vi "LDA_Align_PN.vi"() -> (0 "Beam Data":T1={"Vg1 (Green 1 dir. vect.)"=[0.059117350659853476, -0.996541267827751, 0.05840068807144843], "Vg2  (Green 2 dir. vect.)"=[-0.05232536310393669, -0.9971561380468801, -0.054237373935992664], "Vb1 (Blue 1 dir. vect.)"=[-0.052923229613528855, -0.9969242065933935, 0.057803616456121795], "Vb2 (Blue 1 dir. vect.)"=[0.05971521716944564, -0.9967731992812374, -0.05364030232066602], "Porb (Orb XYZ posn. forced coplanar)"=[2201.0738225655555, -1199.3737231995547, 269.758310600838], "Porb (Orb XYZ posn. - allow skew)"=[2200.796256301178, -1199.3740953152687, 270.0329332816893], "Orb posn. uncertainty, +/- dx, dy, dz"=[0.13878313218879157, 0.00018605785703584843, 0.13731134042564008], "Vp (Actual Probe dir. vect)"=[0.003406702197773746, -0.9999920168246164, 0.0020882210543692924], "Yaw (deg)"=89.80480953887573, "Pitch (deg)"=0.11964634006213794, "In-Plane Roll (deg)"=45.305328966424156, "Beam Half Angle (deg)"=4.544091484248422, "B1 Close P11"=[0.0, 0.0, 0.0], "B1 Far P12"=[2158.01, -491.04, 229.28], "B2 Close P22"=[2158.01, -491.04, 229.28], "B2 Far P21"=[2158.01, -491.04, 229.28], "Projected Roll (deg)"=0.0, "Green Velocity Vector"=[0.0, 0.0, 0.0], "Blue Velocity Vector"=[0.0, 0.0, 0.0], "Probe is facing...."="-", "Calculation Method"=""} {"Vp (Actual Probe dir. vect)" format="%#_6f"; "Vg2  (Green 2 dir. vect.)" format="%#_6f"; "Vg1 (Green 1 dir. vect.)" format="%#_6f"})   [LabVIEW 2011]
uses:
  Controls/LDA_Beam_Cluster.ctl
  Gen Trav/Route mapping/Axis.ctl
  Controls/User_Specific_mode.ctl
  Globals/Constants_global.vi
  Globals/Trav_pos_global.vi
  Globals/LDA_meas_global_1.vi
  Utilities/Email_transfer_global.vi
panel:
  # "Run this Vi again if you taught the laser positions but something went wrong after that"
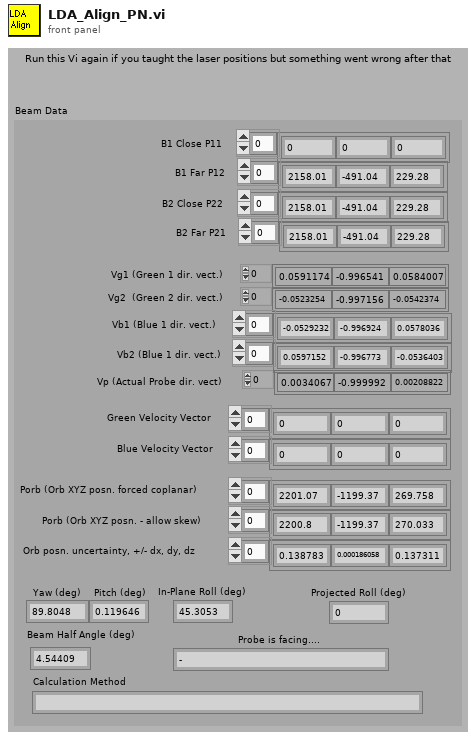
[diagram p1: front panel]
types:
  T1 = typedef "LDA_Beam_Cluster.ctl" = cluster{"Vg1 (Green 1 dir. vect.)":dbl[], "Vg2  (Green 2 dir. vect.)":dbl[], "Vb1 (Blue 1 dir. vect.)":dbl[], "Vb2 (Blue 1 dir. vect.)":dbl[], "Porb (Orb XYZ posn. forced coplanar)":dbl[], "Porb (Orb XYZ posn. - allow skew)":dbl[], "Orb posn. uncertainty, +/- dx, dy, dz":dbl[], "Vp (Actual Probe dir. vect)":dbl[], "Yaw (deg)":dbl, "Pitch (deg)":dbl, "In-Plane Roll (deg)":dbl, "Beam Half Angle (deg)":dbl, "B1 Close P11":dbl[], "B1 Far P12":dbl[], "B2 Close P22":dbl[], "B2 Far P21":dbl[], "Projected Roll (deg)":dbl, "Green Velocity Vector":dbl[], "Blue Velocity Vector":dbl[], "Probe is facing....":string, "Calculation Method":string}
  T2 = typedef "Axis.ctl" = enum16{"X Axis", "X Axis -ve", "Y Axis", "Y Axis -ve", "Z Axis", "Z Axis -ve"}
  T3 = typedef "User_Specific_mode.ctl" = enum16{"Check VI only", "Run VI"}
  T4 = enum16{"Load setup from excel file", "Save setup to excel file"}
  T5 = enum16{"Load From Excel File", "Save to Excel File"}
  T6 = cluster{"second":i32, "minute":i32, "hour":i32, "day of month":i32, "month":i32, "year":i32, "day of week":i32, "day of year":i32, "is DST":i32}
  T7 = typedef "Multi_Run_Status.ctl" = enum16{"Continue", "Jump to Next Point", "Jump to Next Row", "Jump To Fall Back", "Terminate Run"}
  T8 = cluster{"path":path, "data":string, "binary":bool, "MIME content-type \n(application/octet-stream)":string}[]
  T9 = cluster{"path":path, "data":string, "binary":bool, "MIME content-type \n(application/octet-stream)":string}
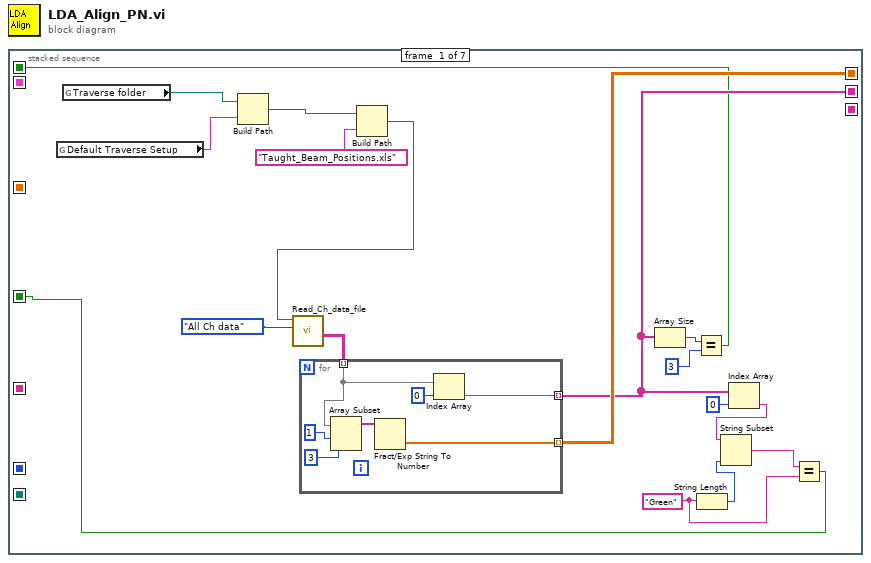
[diagram p0: block diagram]
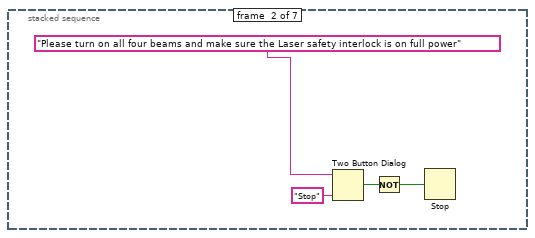
[diagram p2: hidden frame]
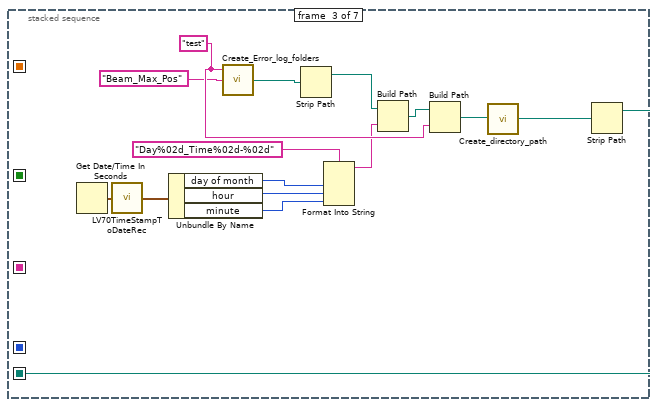
[diagram p3: hidden frame]
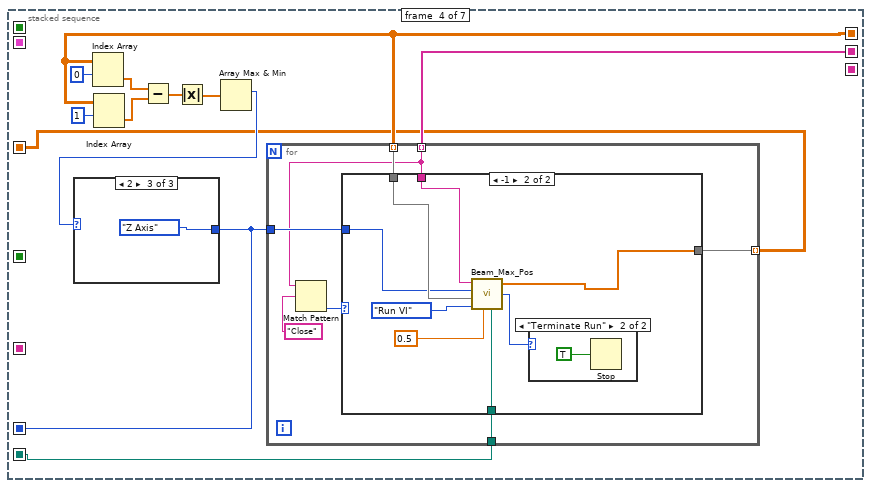
[diagram p4: hidden frame]
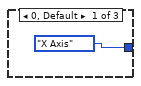
[diagram p5: hidden frame]
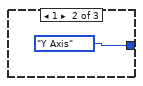
[diagram p6: hidden frame]
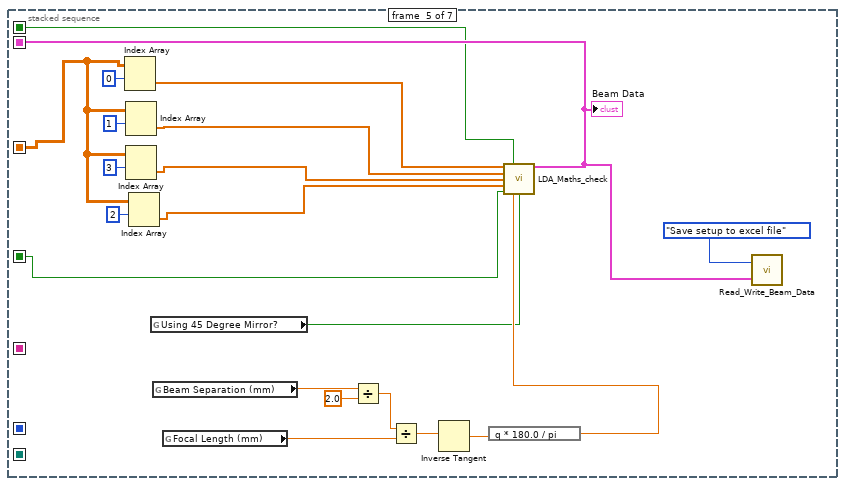
[diagram p9: hidden frame]
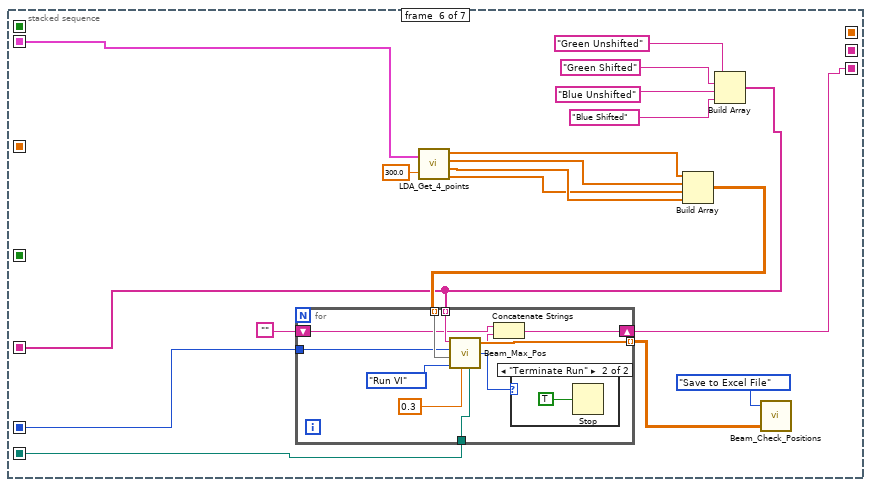
[diagram p10: hidden frame]
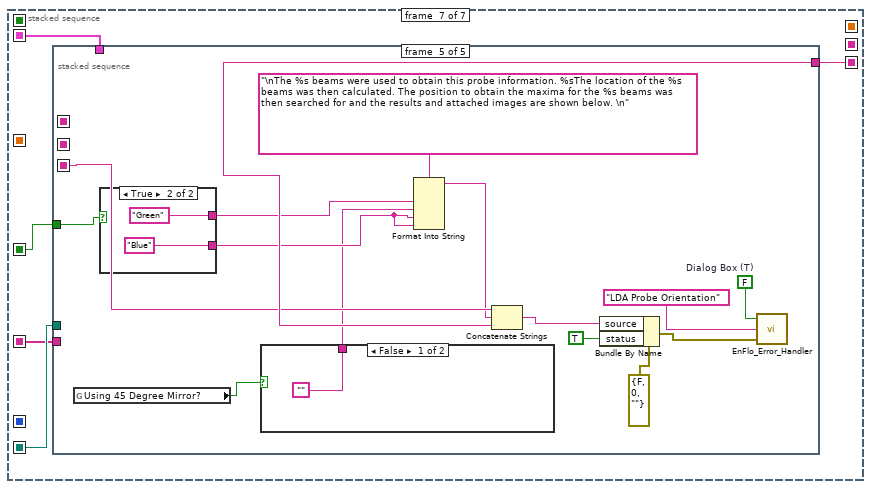
[diagram p12: hidden frame]
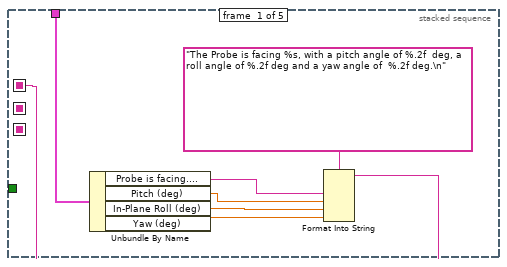
[diagram p13: hidden frame]
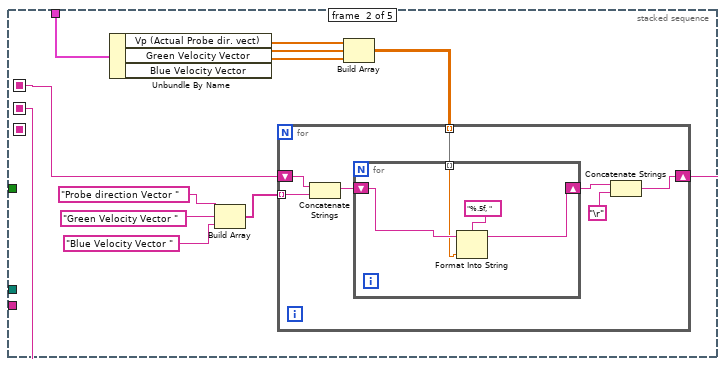
[diagram p14: hidden frame]
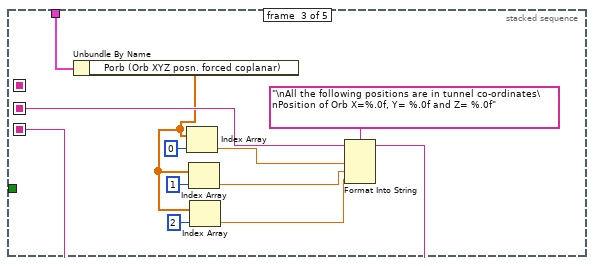
[diagram p15: hidden frame]
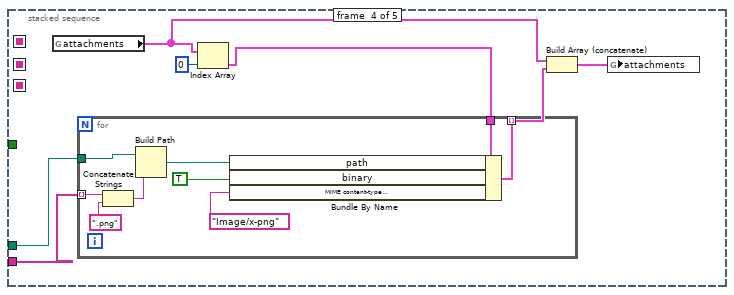
[diagram p16: hidden frame]
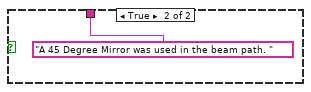
[diagram p17: hidden frame]
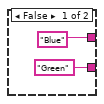
[diagram p18: hidden frame]
diagram:
  n1 = stacked-sequence {
    seq-local: [_ _ _ _ w96 _ _] -> [_ _ _ _ _ w115 w129]
    seq-local: [w12 _ _ _ _ _ _] -> [_ _ _ w53 _ _ _]
    seq-local: [w4 _ _ _ _ _ _] -> [_ _ _ w56 _ _ _]
    seq-local: [_ _ _ w47 _ _ _] -> [_ _ _ _ w84 _ _]
    seq-local: [_ _ w32 _ _ _ _] -> [_ _ _ w46 _ w113 w132]
    seq-local: [_ _ _ w45 _ _ _] -> [_ _ _ _ _ w114 _]
    seq-local: [_ _ _ _ _ w111 _] -> [_ _ _ _ _ _ w131]
    seq-local: [_ _ _ _ _ w109 _] -> [_ _ _ _ _ _ w130]
    seq-local: [w5 _ _ _ _ _ _] -> [_ _ _ _ w78 _ w128]
    seq-local: [w1 _ _ _ _ _ _] -> [_ _ _ _ w77 _ _]
    frame #0 {
      w6 = "Green"
      n2 = global read "Trav_pos_global.vi" "Default Traverse Setup"() -> (w16:string)
      n3 = global read "Constants_global.vi" "Traverse folder"() -> (w18:path)
      n4 = Build Path(base path=w18, name or relative path=w16) -> (appended path=w17:path)
      n5 = Build Path(base path=w17, name or relative path="Taught_Beam_Positions.xls" ("Substring")) -> (appended path=w11:path)
      n6 = call "Read_Ch_data_file.vi"("Output"=enum16{"All Ch data", "The last few rows"}."All Ch data", "Filename"=w11) -> ("Channel Values"=w14:string[][])  [unwired: 3 in, 4 out]
      n7 = for {
        tunnel: w14 -> [w21] mode=indexing
        tunnel: [w23] -> w12 mode=indexing
        tunnel: [w19] -> w4 mode=indexing
        n8 = Array Subset(array=w21, index=1 ("Array Index"), length=3) -> (w24:string[])
        n9 = Fract/Exp String To Number(string=w24) -> (number=w23:dbl[])  [unwired: 4 out]
        n10 = Index Array(array=w21, index=0) -> (element=w19:string)
      }
      n11 = Array Size(array=w4) -> (size(s)=w3:i32)
      n12 = Equal?(x=w3, y=3) -> (x = y?=w1:bool)
      n13 = String Length(string=w6) -> (length=w8:i32)
      n14 = Index Array(array=w4, index=0) -> (element=w9:string)
      n15 = String Subset(string=w9, length (rest)=w8) -> (substring=w7:string)  [unwired: 1 out]
      n16 = Equal?(x=w7, y=w6) -> (x = y?=w5:bool)
    }
    frame #1 {
      n17 = Two Button Dialog(message="Please turn on all four beams and make sure the Laser safety interlock is on full power", 1:"Stop" ("F button name (\"Cancel\")")) -> (T button?=w28:bool)  [unwired: 1 out]
      n18 = Not(x=w28) -> (.not. x?=w27:bool)
      n19 = Stop(stop? (T)=w27) -> ()
    }
    frame #2 {
      w42 = "test" ("Log Filename")
      n20 = Get Date/Time In Seconds() -> (seconds since 1Jan1904=w30:timestamp)
      n21 = call <vilib>:"LV70TimeStampToDateRec.vi"("time stamp"=w30) -> ("date time rec"=w35:T6)
      n22 = Unbundle By Name(w35) -> ("day of month"=w38:i32, "hour"=w37:i32, "minute"=w36:i32)
      n23 = call "Create_Error_log_folders.vi"("Log Folder"="Beam_Max_Pos" ("name or relative path"), "Log Filename"=w42) -> ("Server copy Location"=w31:path)  [unwired: 1 in, 2 out]
      n24 = Strip Path(path=w31) -> (stripped path=w34:path)  [unwired: 1 out]
      n25 = Format Into String(format string="Day%02d_Time%02d-%02d", w38, w37, w36) -> (resulting string=w33:string)  [unwired: 2 in, 1 out]
      n26 = Build Path(base path=w34, name or relative path=w33) -> (appended path=w41:path)
      n27 = Build Path(base path=w41, name or relative path=w42) -> (appended path=w43:path)
      n28 = call "Create_directory_path.vi"("Path name"=w43) -> ("Path name Out"=w44:path)  [unwired: 1 in, 1 out]
      n29 = Strip Path(path=w44) -> (stripped path=w32:path)  [unwired: 1 out]
    }
    frame #3 {
      n30 = Index Array(array=w53, index (row)=0) -> (element=w52:dbl[])  [unwired: 1 in]
      n31 = Index Array(array=w53, index (row)=1) -> (element=w51:dbl[])  [unwired: 1 in]
      n32 = Subtract(x=w52, y=w51) -> (x-y=w50:dbl[])
      n33 = Absolute Value(x=w50) -> (abs(x)=w49:dbl[])
      n34 = Array Max & Min(array=w49) -> (max index (indices)=w48:i32)  [unwired: 3 out]
      n35 = case shown="2" w48 {
        tunnel: [Axis."X Axis" ("Fixed Axis") Axis."Y Axis" ("Fixed Axis") Axis."Z Axis" ("Fixed Axis")] -> w45
        frame 0, Default {
        }
        frame 1 {
        }
        frame 2 {
        }
      }
      n36 = for {
        tunnel: w56 -> [w62] mode=indexing
        tunnel: w53 -> [w66] mode=indexing
        tunnel: w45 -> [w65]
        tunnel: w46 -> [w64]
        tunnel: [w63] -> w47 mode=indexing
        n37 = Match Pattern(string=w62, regular expression="Close") -> (offset past match=w60:i32)  [unwired: 4 out]
        n38 = case shown="-1" w60 {
          tunnel: w62 -> [_ w75]
          tunnel: w66 -> [w67 w74]
          tunnel: w65 -> [_ w72]
          tunnel: w64 -> [_ w71]
          tunnel: [w67 w70] -> w63
          frame 0, Default {
          }
          frame -1 {
            n39 = call "Beam_Max_Pos.vi"("Picture Log"=w71, "Search Step (mm)"=0.5, "Mode"=User_Specific_mode."Run VI", "Starting Position"=w74, "Fixed Axis"=w72, "Beam Name"=w75) -> ("Status"=w68:T7, "Beam maxima"=w70:dbl[])  [unwired: 1 in, 2 out]
            n40 = case shown="\"Terminate Run\"" w68 {
              frame "Continue", Default {
              }
              frame "Terminate Run" {
                n41 = Stop(stop? (T)=TRUE) -> ()
              }
            }
          }
        }
      }
    }
    frame #4 {
      n42 = Index Array(array=w84, index (row)=0) -> (element=w83:dbl[])  [unwired: 1 in]
      n43 = Index Array(array=w84, index (row)=1) -> (element=w82:dbl[])  [unwired: 1 in]
      n44 = Index Array(array=w84, index (row)=3) -> (element=w81:dbl[])  [unwired: 1 in]
      n45 = Index Array(array=w84, index (row)=2) -> (element=w80:dbl[])  [unwired: 1 in]
      n46 = global read "LDA_meas_global_1.vi" "Using 45 Degree Mirror?"() -> (w79:bool)
      n47 = global read "LDA_meas_global_1.vi" "Beam Separation (mm)"() -> (w95:dbl)
      n48 = global read "LDA_meas_global_1.vi" "Focal Length (mm)"() -> (w92:dbl)
      n49 = Divide(x=w95, y=2.0) -> (x/y=w93:dbl)
      n50 = Divide(x=w93, y=w92) -> (x/y=w90:dbl)
      n51 = Inverse Tangent(1:w90) -> (0:w91:dbl)
      n52 = expression code="q * 180.0 / pi"(w91) -> (w89:dbl)
      n53 = call "LDA_Maths_check.vi"("B1 Close P11"=w83, "Use Specification Beam Half-Angle"=w77, "B1 Far P12"=w82, "B2 Close P22"=w81, "B2 Far P21"=w80, "Use Green Beams (True) or Blue Beams (False)"=w78, "Beam Half-Angle (deg)"=w89, "Using 45 Degree Mirror?"=w79) -> ("Beam Data"=w96:T1)  [unwired: 7 out]
      "Beam Data" <- w96
      n54 = call "Read_Write_Beam_Data.vi"("Beam Data In"=w96, "Mode"=T4."Save setup to excel file") -> ()  [unwired: 1 out]
    }
    frame #5 {
      n55 = call "LDA_Get_4_points.vi"("Beam Data"=w115, "L, Probe-Normal Distance"=300.0) -> ("Pg1"=w103:dbl[], "Pg2"=w102:dbl[], "Pb1"=w99:dbl[], "Pb2"=w98:dbl[])
      n56 = Build Array(w103, w102, w98, w99) -> (w112:dbl[][])
      n57 = Build Array("Green Unshifted", "Green Shifted", "Blue Unshifted", "Blue Shifted") -> (w111:string[])
      n58 = for {
        tunnel: w112 -> [w125] mode=indexing
        tunnel: w114 -> [w124]
        tunnel: w113 -> [w123]
        tunnel: [w122] -> w100 mode=indexing
        tunnel: w111 -> [w121] mode=indexing
        shift-right: [w118] -> w109
        shift-left: "" -> [w120]
        n59 = call "Beam_Max_Pos.vi"("Picture Log"=w123, "Search Step (mm)"=0.3, "Mode"=User_Specific_mode."Run VI", "Starting Position"=w125, "Fixed Axis"=w124, "Beam Name"=w121) -> ("Status"=w116:T7, "Beam maxima"=w122:dbl[], "Message"=w119:string)  [unwired: 1 in, 1 out]
        n60 = Concatenate Strings(w120, w119) -> (w118:string)
        n61 = case shown="\"Terminate Run\"" w116 {
          frame "Continue", Default {
          }
          frame "Terminate Run" {
            n62 = Stop(stop? (T)=TRUE) -> ()
          }
        }
      }
      n63 = call "Beam_Check_Positions.vi"("Values"=w100, "Mode"=T5."Save to Excel File") -> ()  [unwired: 2 out]
    }
    frame #6 {
      n64 = stacked-sequence {
        seq-local: [w133 _ _ _ _] -> [_ w141 _ _ _]
        seq-local: [_ w140 _ _ _] -> [_ _ w171 _ _]
        seq-local: [_ _ w162 _ _] -> [_ _ _ _ w196]
        tunnel: w132 -> [_ _ _ w174 _]
        tunnel: w131 -> [_ _ _ w173 _]
        tunnel: w130 -> [_ _ _ _ w198]
        tunnel: w129 -> [w139 w150 w172 _ _]
        tunnel: w128 -> [_ _ _ _ w195]
        frame #0 {
          n65 = Unbundle By Name(w139) -> ("Probe is facing...."=w138:string, "Pitch (deg)"=w137:dbl, "In-Plane Roll (deg)"=w136:dbl, "Yaw (deg)"=w135:dbl)
          n66 = Format Into String(format string="The Probe is facing %s, with a pitch angle of %.2f  deg, a roll angle of %.2f deg and a yaw angle of  %.2f deg.\n", w138, w137, w136, w135) -> (resulting string=w133:string)  [unwired: 2 in, 1 out]
        }
        frame #1 {
          n67 = Unbundle By Name(w150) -> ("Vp (Actual Probe dir. vect)"=w145:dbl[], "Green Velocity Vector"=w144:dbl[], "Blue Velocity Vector"=w143:dbl[])
          n68 = Build Array("Probe direction Vector ", "Green Velocity Vector ", "Blue Velocity Vector ") -> (w146:string[])
          n69 = Build Array(w145, w144, w143) -> (w142:dbl[][])
          n70 = for {
            shift-right: [w152] -> w140
            shift-left: w141 -> [w155]
            tunnel: w146 -> [w154] mode=indexing
            tunnel: w142 -> [w151] mode=indexing
            n71 = Concatenate Strings(w155, w154) -> (w153:string)
            n72 = for {
              shift-right: [w159] -> w156
              shift-left: w153 -> [w160]
              tunnel: w151 -> [w158] mode=indexing
              n73 = Format Into String(format string="%.5f, " ("Format String"), initial string=w160, w158) -> (resulting string=w159:string)  [unwired: 1 in, 1 out]
            }
            n74 = Concatenate Strings(w156, "\r") -> (w152:string)
          }
        }
        frame #2 {
          n75 = Unbundle By Name(w172) -> ("Porb (Orb XYZ posn. forced coplanar)"=w167:dbl[])
          n76 = Index Array(array=w167, index=0) -> (element=w166:dbl)
          n77 = Index Array(array=w167, index=1) -> (element=w165:dbl)
          n78 = Index Array(array=w167, index=2) -> (element=w164:dbl)
          n79 = Format Into String(format string="\nAll the following positions are in tunnel co-ordinates\nPosition of Orb X=%.0f, Y= %.0f and Z= %.0f", initial string=w171, w166, w165, w164) -> (resulting string=w162:string)  [unwired: 1 in, 1 out]
        }
        frame #3 {
          n80 = global read "Email_transfer_global.vi" "attachments"() -> (w177:T8)
          n81 = Index Array(array=w177, index=0) -> (element=w176:T9)
          n82 = for {
            tunnel: [w186] -> w179 mode=indexing
            tunnel: w176 -> [w185]
            tunnel: w174 -> [w183]
            tunnel: w173 -> [w181] mode=indexing
            n83 = Concatenate Strings(w181, ".png" ("string")) -> (w180:string)
            n84 = Build Path(base path=w183, name or relative path=w180) -> (appended path=w184:path)
            n85 = Bundle By Name(cluster=w185, "path"=w184, "binary"=TRUE, "MIME content-type \n(application/octet-stream)"="Image/x-png" ("MIME content-type \n(application/octet-stream)")) -> (w186:T9)
          }
          n86 = Build Array (concatenate)(w177, w179) -> (w178:T8)
          n87 = global write "Email_transfer_global.vi" "attachments"(w178) -> ()
        }
        frame #4 {
          w202 = FALSE  # Dialog Box (T)
          n88 = global read "LDA_meas_global_1.vi" "Using 45 Degree Mirror?"() -> (w190:bool)
          n89 = case shown="True" w195 {
            tunnel: ["Green" "Blue"] -> w192
            tunnel: ["Blue" "Green"] -> w193
            frame False {
            }
            frame True {
            }
          }
          n90 = case shown="False" w190 {
            tunnel: ["" "A 45 Degree Mirror was used in the beam path. "] -> w189
            frame False {
            }
            frame True {
            }
          }
          n91 = Format Into String(format string="\nThe %s beams were used to obtain this probe information. %sThe location of the %s beams was then calculated. The position to obtain the maxima for the %s beams was then searched for and the results and attached images are shown below. \n", w193, w189, w192, w192) -> (resulting string=w191:string)  [unwired: 2 in, 1 out]
          n92 = Concatenate Strings(w196, w191, w198) -> (w197:string)
          n93 = Bundle By Name(cluster=errorcluster {"status"=FALSE, "code"=0, "source"=""} ("error in (no error)"), "source"=w197, "status"=TRUE ("Bundle Element")) -> (w200:errorcluster)
          n94 = call "EnFlo_Error_Handler.vi"("error in (no error)"=w200, "Error Type"="LDA Probe Orientation", "Dialog Box (T)"=w202) -> ()  [unwired: 3 out]
        }
      }
    }
  }
